vi "GOLPI Update State Display.vi"(7 "stat ref":refnum<vi>, 8 "error in":errorcluster, 11 "golpi ref":refnum<vi>) -> (0 "error out":errorcluster)   [LabVIEW 2020]
doc: "Updates GOLPI state display based on GOLPI running check and exclusive access semaphore state (stopped, ready, busy). Provide reference to state indicator. Call periodically ideally in separate thread."
uses:
  golpi_session.ctl
  GOLPI reference Type Def.ctl
  Pipe Handle.ctl
  varilib/SGUI Assign Single String With Tags.vi
  GOLPI Multi Process.lvlib
  varilib/varilib.lvlib
  LV Process library.lvlib
  GOLPI library.lvlib
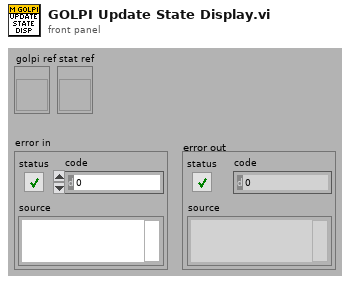
[diagram p1: front panel]
types:
  T1 = typedef "GOLPI library.lvlib/GOLPI reference Type Def.ctl" = cluster{"pipe handle":T2, "fast read timeout [ms]":u32, "fast read settle time [ms]":u32, "fast read to multiple [ms]":u32, "max elements per input line":u32, "slow read timeout [ms]":u32, "stdin double format specifier":string, "max elements per stdout output column":u32, "console mode bitstream":bool, "bitstream first read timeout [ms]":u32, "bitstream read timeout [ms]":u32, "struct transfer possible":bool, "matlab mode":bool}
  T2 = typedef "LV Process library.lvlib/Pipe Handle.ctl" = cluster{"lv_proc.dll file path":path, "process instance handle":u32[], "debug mode":bool, "debug data":cluster{"time":timestamp, "stdin":bool, "data":string}[]}
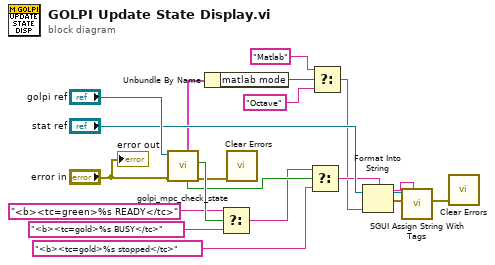
[diagram p0: block diagram]
diagram:
  n1 = call "golpi_mpc_check_state.vi"("error in"="error in", "golpi session ref"="golpi ref") -> ("error out"=w17:errorcluster, "GOLPI ready?"=w19:bool, "GOLPI running?"=w16:bool, "GOLPI ref"=w9:T1)  [unwired: 4 in, 2 out]
  n2 = Unbundle By Name(w9) -> ("matlab mode"=w8:bool)
  n3 = Select(t="<b><tc=green>%s READY</tc>", s=w19, f="<b><tc=gold>%s BUSY</tc>") -> (s? t:f=w14:string)
  n4 = call <vilib>:"Clear Errors.vi"("error in (no error)"=w17) -> ()  [unwired: 5 in, 2 out]
  n5 = Select(t=w14, s=w16, f="<b><tc=gold>%s stopped</tc>") -> (s? t:f=w4:string)
  n6 = Select(t="Matlab", s=w8, f="Octave") -> (s? t:f=w3:string)
  n7 = Format Into String(format string=w4, w3) -> (resulting string=w1:string, error out=w5:errorcluster)  [unwired: 2 in]
  n8 = call-poly "SGUI Assign String With Tags.vi"("error in"=w5, "string ref"="stat ref", "string (empty)"=w1) -> ("error out"=w2:errorcluster)  [unwired: 7 in, 1 out]
  n9 = call <vilib>:"Clear Errors.vi"("error in (no error)"=w2) -> ()  [unwired: 5 in, 2 out]
  "error out" <- "error in"
